vi "Main.vi"(8 "error in":errorcluster, 11 "Philosopher in":refnum<class "Philosopher.lvclass">) -> (0 "error out":errorcluster, 3 "Philosopher out":refnum<class "Philosopher.lvclass">)   [LabVIEW 2021, in "Philosopher.lvclass"]
doc: "The <b>Queued Message Handler</b> of the Worker that owns this VI."
uses:
  Philosopher.lvclass
  Philosopher.lvclass/Philosopher.ctl
  Initialization Data.ctl
  Response Cases.ctl
  <vilib>/Utility/miscctls.llb/LVRectTypeDef.ctl
  <vilib>/addons/_Workers/Library/Case Label.ctl
  <vilib>/addons/_Workers/Library/Workers.lvlib
  Utility/Utility.lvlib
  Timer/Timer.lvclass
panel:
  out "time eating [s]":dbl format="%.1f"
  out "ID":i32
  out "State Picture":u16(ring)
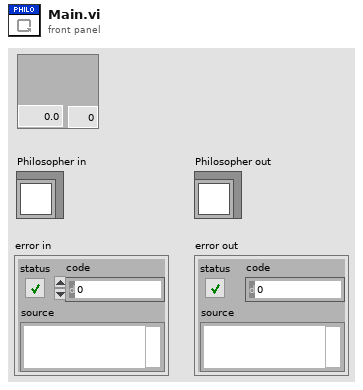
[diagram p1: front panel]
types:
  T1 = typedef "Philosopher.lvclass/Initialization Data.ctl" = cluster{"Response Cases":T2, "ID":i32, "FP.PanelBounds":T4}
  T2 = typedef "Philosopher.lvclass/Response Cases.ctl" = cluster{"Hungry":T3, "Done":T3}
  T3 = typedef "Workers.lvlib/Case Label.ctl" = string
  T4 = typedef "LVRectTypeDef.ctl" = cluster{"Left":i16, "Top":i16, "Right":i16, "Bottom":i16}
  T5 = enum16{"initial", "thinking", "hungry", "eating"}
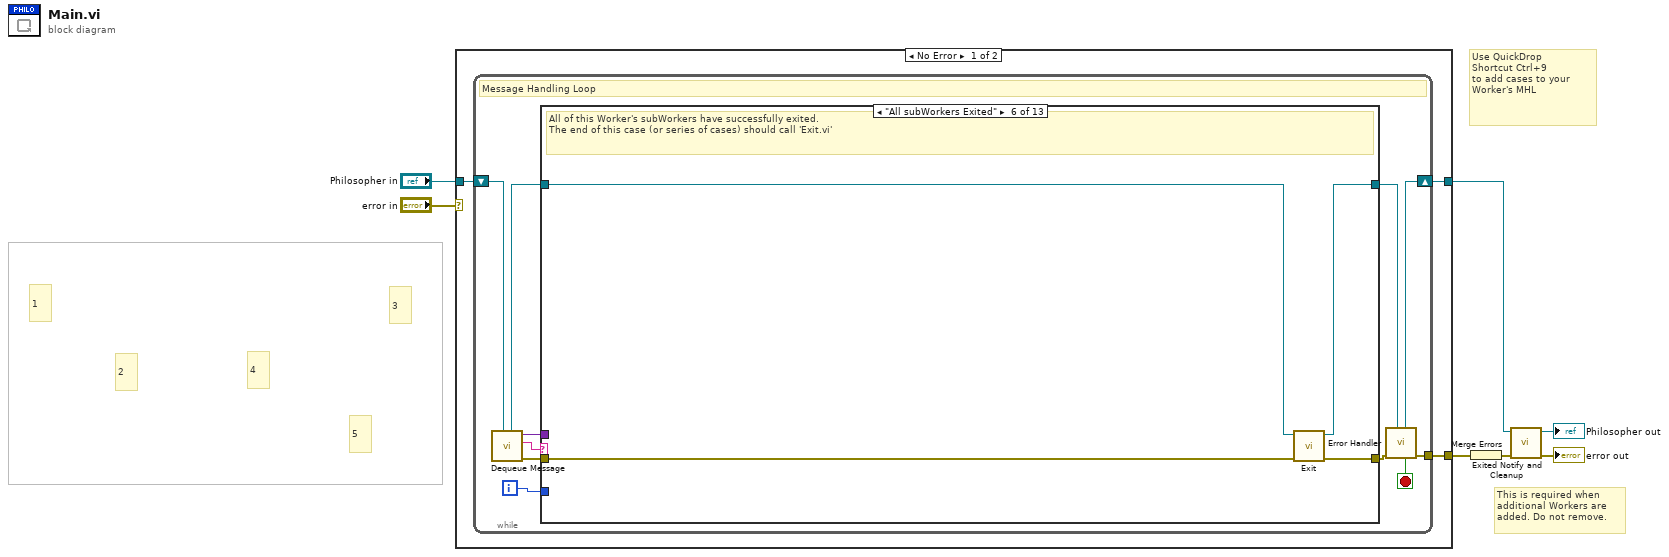
[diagram p0: block diagram]
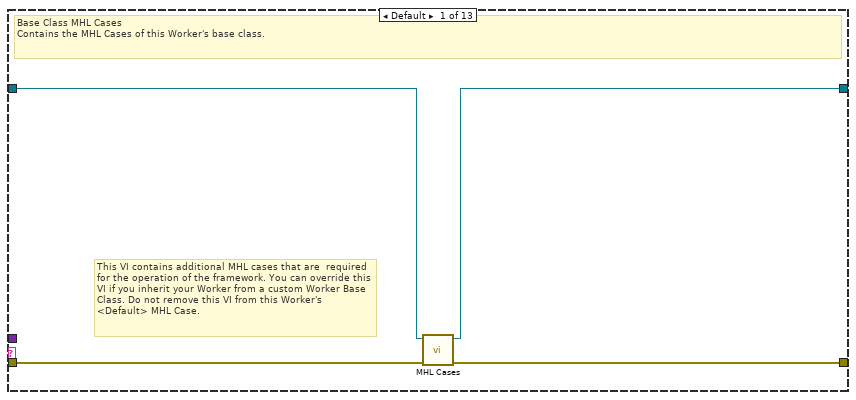
[diagram p2: hidden frame]
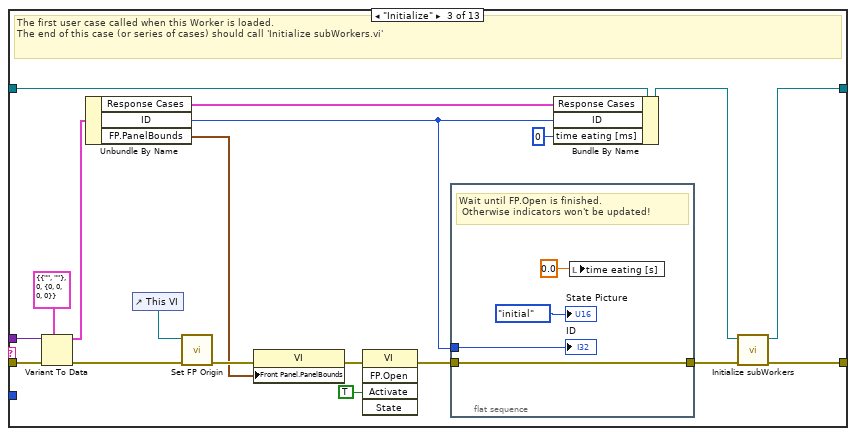
[diagram p4: hidden frame]
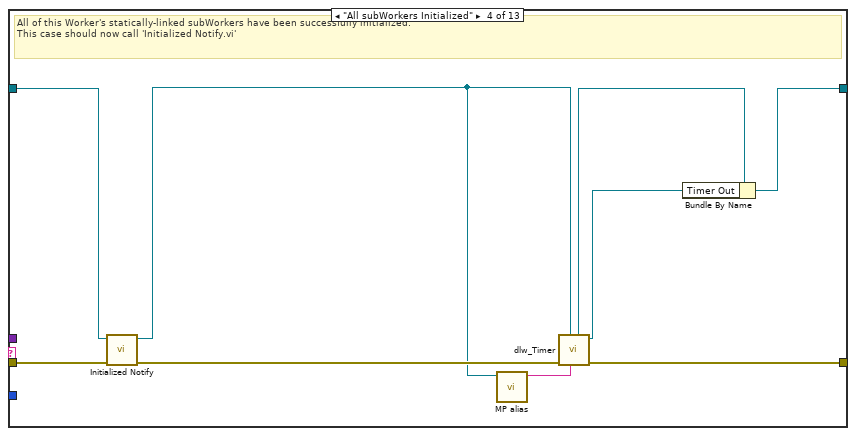
[diagram p5: hidden frame]
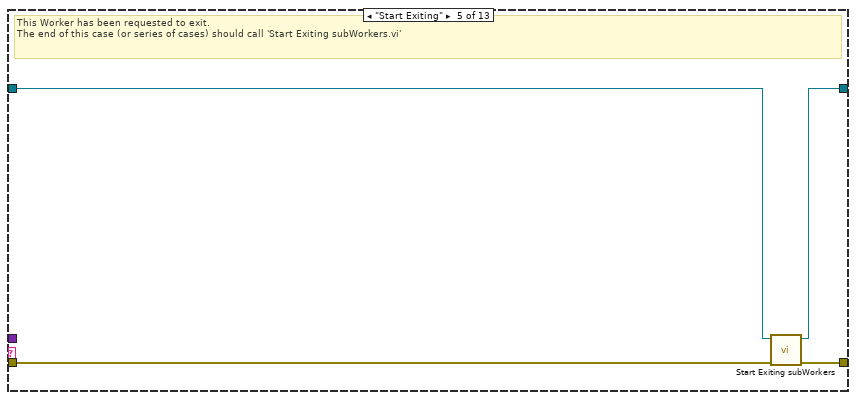
[diagram p6: hidden frame]
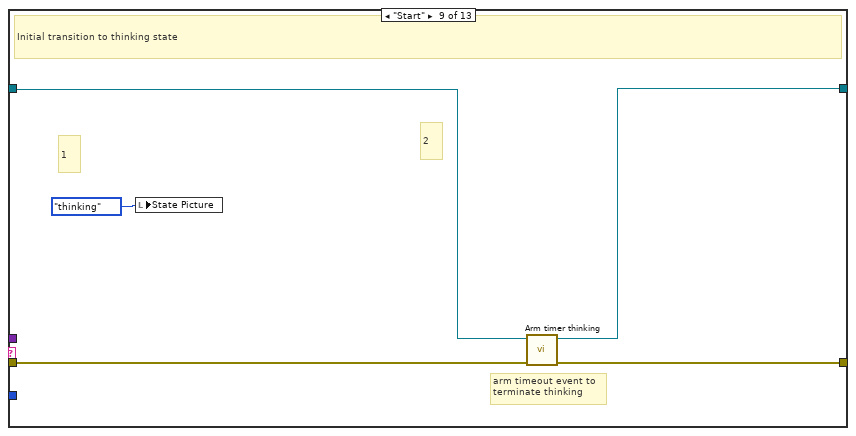
[diagram p9: hidden frame]
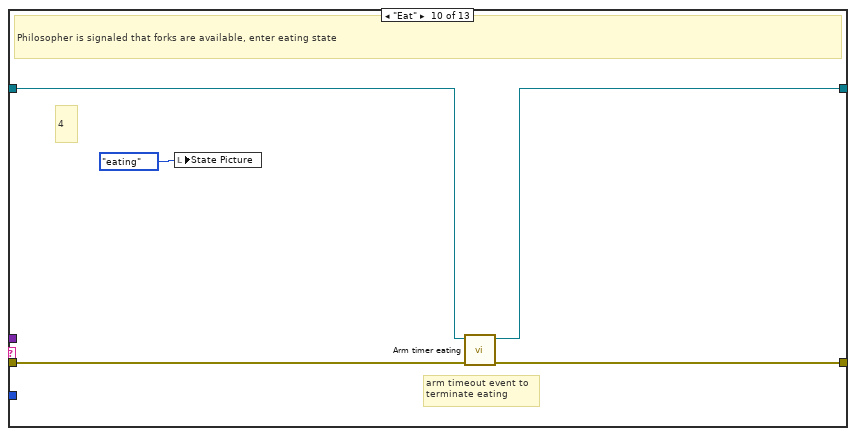
[diagram p10: hidden frame]
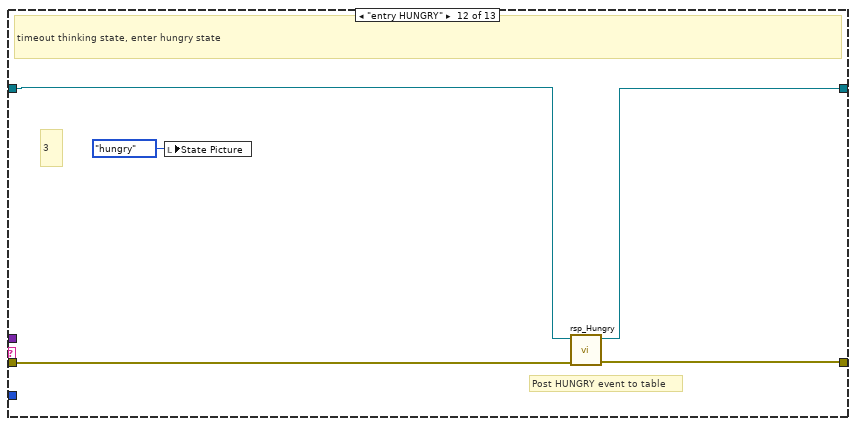
[diagram p12: hidden frame]
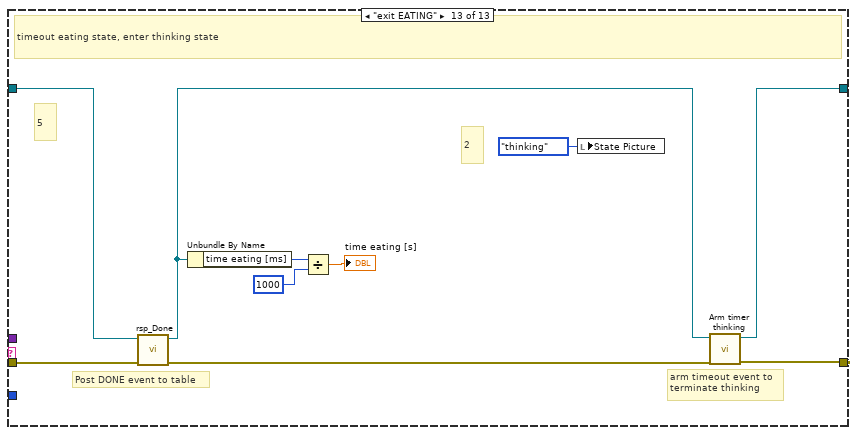
[diagram p13: hidden frame]
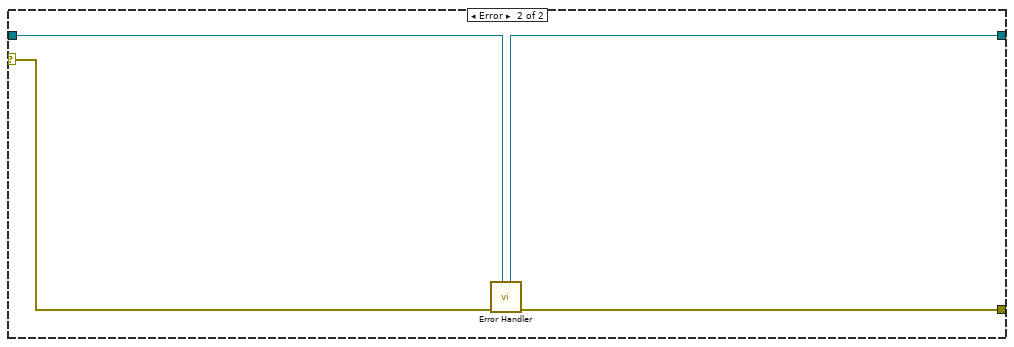
[diagram p14: hidden frame]
diagram:
  # "3"
  # "2"
  # "5"
  # "4"
  # "1"
  # "Use QuickDrop\nShortcut Ctrl+9\nto add cases to your\nWorker's MHL"
  # "This is required when additional Workers are added. Do not remove."
  n1 = case shown="No Error" "error in" {
    tunnel: "Philosopher in" -> [w8 w100]
    tunnel: [w10 w101] -> w6
    tunnel: [w9 w99] -> w7
    selector: "error in" -> [_ w102]
    frame No Error {
      n2 = while {
        shift-right: [w19] -> w9
        shift-left: w8 -> [w21]
        tunnel: [w20] -> w10
        i -> [w12]
        stop <- w13 stop-if-true
        # "Message Handling Loop"
        n3 = call-dynamic "Dequeue Message.vi"("Worker"=w21) -> ("error out"=w18:errorcluster, "Case out"=w14:string, "Data out"=w11:variant, "Worker out"=w16:refnum<class "Philosopher.lvclass">)  [unwired: 6 in, 1 out]
        n4 = case "Worker MHL Case Structure (DO NOT CHANGE LABEL NAME)" shown="\"All subWorkers Exited\"" w14 {
          tunnel: w18 -> [w25 w26 w44 w59 w60 w67 w69 w71 w74 w81 w83 w87 w92]
          tunnel: [w24 w26 w46 w56 w63 w66 w69 w71 w76 w78 w83 w85 w93] -> w17
          tunnel: w16 -> [w23 w27 w43 w58 w61 w65 w68 w70 w72 w80 w82 w86 w91]
          tunnel: [w22 w27 w45 w53 w62 w64 w68 w70 w75 w77 w82 w84 w90] -> w15
          tunnel: w12 -> [_ _ _ _ _ _ _ _ _ _ _ _ _]
          tunnel: w11 -> [_ _ w42 _ _ _ _ _ _ _ _ _ _]
          frame Default {
            # "This VI contains additional MHL cases that are  required for the operation of the framework. You can override this VI if you inherit your Worker from a custom Worker Base Class. Do not remove this VI from this Worker's <Default> MHL Case."
            # "Base Class MHL Cases\nContains the MHL Cases of this Worker's base class."
            n5 = call-dynamic "MHL Cases.vi"("error in"=w25, "Worker in"=w23) -> ("error out"=w24:errorcluster, "Worker out"=w22:refnum<class "Philosopher.lvclass">)  [unwired: 8 in]
          }
          frame "------------ FRAMEWORK CASES -----------" {
            # "Start of Workers Framework Cases"
          }
          frame "Initialize" {
            # "The first user case called when this Worker is loaded.\nThe end of this case (or series of cases) should call 'Initialize subWorkers.vi'"
            n6 = Variant To Data(error in=w44, type=T1 {"Response Cases"={"Hungry"="", "Done"=""}, "ID"=0, "FP.PanelBounds"={"Left"=0, "Top"=0, "Right"=0, "Bottom"=0}} ("Cluster"), Variant=w42) -> (data=w40:T1, error out=w32:errorcluster)
            n7 = Unbundle By Name(w40) -> ("Response Cases"=w39:T2, "ID"=w34:i32, "FP.PanelBounds"=w29:T4)
            n8 = control-ref of="This VI"() -> (w30:refnum<vi>)
            n9 = call "Set FP Origin.vi"("error in"=w32, "VI ref in"=w30) -> ("error out"=w31:errorcluster)  [unwired: 8 in, 1 out]
            n10 = property on="Property Node" class="VI"(error in=w31, "Front Panel.PanelBounds"=w29) -> (error out=w37:errorcluster)  [unwired: 1 in, 1 out]
            n11 = invoke on="Invoke Node" class="VI" method="FP.Open"(error in=w37, "Activate"=TRUE ("Activate?")) -> (error out=w36:errorcluster)  [unwired: 3 in, 4 out]
            n12 = flat-sequence {
              tunnel: [w50] -> w35
              tunnel: w36 -> [w50]
              tunnel: w34 -> [w49]
              frame #0 {
                # "Wait until FP.Open is finished.\n Otherwise indicators won't be updated!"
                n13 = local write "time eating [s]"(0.0 ("time eating")) -> ()
                "State Picture" <- T5."initial" ("State")
                "ID" <- w49
              }
            }
            n14 = Bundle By Name(cluster=w43, "Response Cases"=w39, "ID"=w34, "time eating [ms]"=0) -> (w41:refnum<class "Philosopher.lvclass">)
            n15 = call-dynamic "Initialize subWorkers.vi"("error in"=w35, "Worker"=w41) -> ("error out"=w46:errorcluster, "dup Worker out"=w45:refnum<class "Philosopher.lvclass">)  [unwired: 8 in]
          }
          frame "All subWorkers Initialized" {
            # "All of this Worker's statically-linked subWorkers have been successfully initialized.\nThis case should now call 'Initialized Notify.vi'"
            n16 = call-dynamic "Initialized Notify.vi"("error in"=w59, "Worker"=w58) -> ("error out"=w57:errorcluster, "dup Worker out"=w55:refnum<class "Philosopher.lvclass">)  [unwired: 8 in]
            n17 = call "MP alias.vi"("Philosopher in"=w55) -> ("MP Alias"=w51:string)  [unwired: 10 in]
            n18 = call "dlw_Timer.vi"("Worker Alias"=w51, "Caller in"=w55, "error in"=w57) -> ("error out"=w56:errorcluster, "Timer Out"=w52:refnum<class "Timer.lvclass">, "dup Caller out"=w54:refnum<class "Philosopher.lvclass">)  [unwired: 6 in]
            n19 = Bundle By Name(cluster=w54, "Timer Out"=w52) -> (w53:refnum<class "Philosopher.lvclass">)
          }
          frame "Start Exiting" {
            # "This Worker has been requested to exit. \nThe end of this case (or series of cases) should call 'Start Exiting subWorkers.vi'"
            n20 = call-dynamic "Start Exiting subWorkers.vi"("error_in"=w60, "Worker"=w61) -> ("error out"=w63:errorcluster, "dup Worker out"=w62:refnum<class "Philosopher.lvclass">)  [unwired: 8 in]
          }
          frame "All subWorkers Exited" {
            # "All of this Worker's subWorkers have successfully exited. \nThe end of this case (or series of cases) should call 'Exit.vi'"
            n21 = call-dynamic "Exit.vi"("error_in"=w67, "Worker"=w65) -> ("error out"=w66:errorcluster, "dup Worker out"=w64:refnum<class "Philosopher.lvclass">)  [unwired: 8 in]
          }
          frame "------------- LOCAL API CASES -------------" {
            # "Start of Workers Local API Cases"
          }
          frame "------------- PUBLIC API CASES -------------" {
            # "Start of Workers Public API Cases"
          }
          frame "Start" {
            # "2"
            # "1"
            # "arm timeout event to\nterminate thinking"
            # "Initial transition to thinking state"
            n22 = local write "State Picture"(T5."thinking" ("State")) -> ()
            n23 = call "Arm timer thinking.vi"("error in"=w74, "Philosopher in"=w72) -> ("error out"=w76:errorcluster, "Philosopher out"=w75:refnum<class "Philosopher.lvclass">)  [unwired: 8 in]
          }
          frame "Eat" {
            # "4"
            # "arm timeout event to\nterminate eating"
            # "Philosopher is signaled that forks are available, enter eating state"
            n24 = local write "State Picture"(T5."eating" ("State")) -> ()
            n25 = call "Arm timer eating.vi"("error in"=w81, "Philosopher in"=w80) -> ("error out"=w78:errorcluster, "Philosopher out"=w77:refnum<class "Philosopher.lvclass">)  [unwired: 8 in]
          }
          frame "------------- RESPONSE CASES --------------" {
            # "Start of Workers Response Cases"
          }
          frame "entry HUNGRY" {
            # "3"
            # "Post HUNGRY event to table"
            # "timeout thinking state, enter hungry state"
            n26 = local write "State Picture"(T5."hungry" ("State")) -> ()
            n27 = call "rsp_Hungry.vi"("error in"=w87, "Philosopher in"=w86) -> ("error out"=w85:errorcluster, "dup Philosopher out"=w84:refnum<class "Philosopher.lvclass">)  [unwired: 8 in]
          }
          frame "exit EATING" {
            # "5"
            # "2"
            # "arm timeout event to\nterminate thinking"
            # "Post DONE event to table"
            # "timeout eating state, enter thinking state"
            n28 = call "rsp_Done.vi"("error in"=w92, "Philosopher in"=w91) -> ("error out"=w98:errorcluster, "dup Philosopher out"=w89:refnum<class "Philosopher.lvclass">)  [unwired: 8 in]
            n29 = Unbundle By Name(w89) -> ("time eating [ms]"=w97:i32)
            n30 = Divide(x=w97, y=1000) -> (x/y=→"time eating [s]":dbl)
            n31 = local write "State Picture"(T5."thinking" ("State")) -> ()
            n32 = call "Arm timer thinking.vi"("error in"=w98, "Philosopher in"=w89) -> ("error out"=w93:errorcluster, "Philosopher out"=w90:refnum<class "Philosopher.lvclass">)  [unwired: 8 in]
          }
        }
        n33 = call-dynamic "Error Handler.vi"("Worker"=w15, "error_in"=w17) -> ("error out"=w20:errorcluster, "Stop Loop"=w13:bool, "Worker out"=w19:refnum<class "Philosopher.lvclass">)  [unwired: 7 in]
      }
    }
    frame Error {
      n34 = call-dynamic "Error Handler.vi"("Worker"=w100, "error_in"=w102) -> ("error out"=w101:errorcluster, "Worker out"=w99:refnum<class "Philosopher.lvclass">)  [unwired: 7 in, 1 out]
    }
  }
  n35 = Merge Errors(w6) -> (w3:errorcluster)
  n36 = call-dynamic "Exited Notify and Cleanup.vi"("error_in"=w3, "Worker"=w7) -> ("error out"=→"error out":errorcluster, "dup Worker out"=→"Philosopher out":refnum<class "Philosopher.lvclass">)  [unwired: 8 in]
